vi "Main.vi"(8 "error in":errorcluster, 11 "CPU Percent in":refnum<class "CPU Percent.lvclass">) -> (0 "error out":errorcluster, 3 "CPU Percent out":refnum<class "CPU Percent.lvclass">)   [LabVIEW 2024, in "CPU Percent.lvclass"]
doc: "The <b>Queued Message Handler</b> of the Worker that owns this VI."
uses:
  CPU Percent.lvclass
  C:/Program Files (x86)/National Instruments/LabVIEW 2024/vi.lib/addons/_Workers/Library/Classes/Worker/Worker.lvclass
  CPU Percent.lvclass/CPU Percent.ctl
  rwr_Get CPU Percent Reply.ctl
  Controller/Controller.lvclass
  <vilib>/Analysis/baseanly.llb/Mean (DBL).vi
  <vilib>/Python/Open Venv Python Session.vi
  <vilib>/addons/_Workers/Library/Classes/Worker/Worker.lvclass
  <vilib>/addons/_Workers/Library/Classes/Message Queue/Message Queue.lvclass
  <vilib>/Analysis/NI_AALBase.lvlib
  Initialization Data.ctl
  C:/Program Files (x86)/National Instruments/LabVIEW 2024/vi.lib/addons/_Workers/Library/Classes/Workers Object/Workers Object.lvclass
  C:/_Repo/ugm24-dp2/src/Workers/CPU Percent/CPU Percent.lvclass
panel:
  out "CPU Core Percent":dbl[](array[numeric])
  out "Percent":dbl
  in  "GetPercent":bool
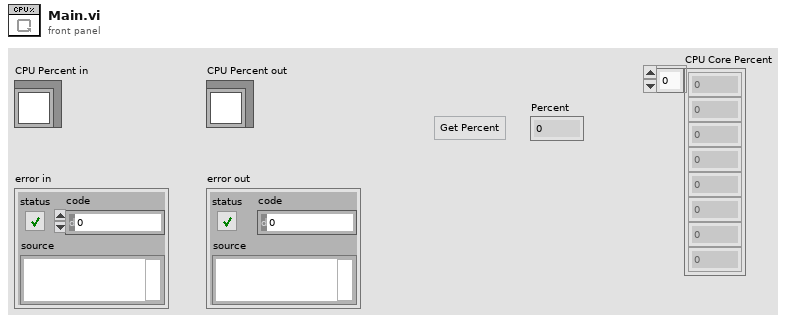
[diagram p1: front panel]
types:
  T1 = typedef "CPU Percent.lvclass/Initialization Data.ctl" = cluster{"String":string, "Show Frontpanel":bool}
  T2 = enum32{"Invalid", "Standard", "Closed", "Hidden", "Minimized", "Maximized"}
  T3 = typedef "CPU Percent.lvclass/rwr_Get CPU Percent Reply.ctl" = cluster{"Percent":dbl}
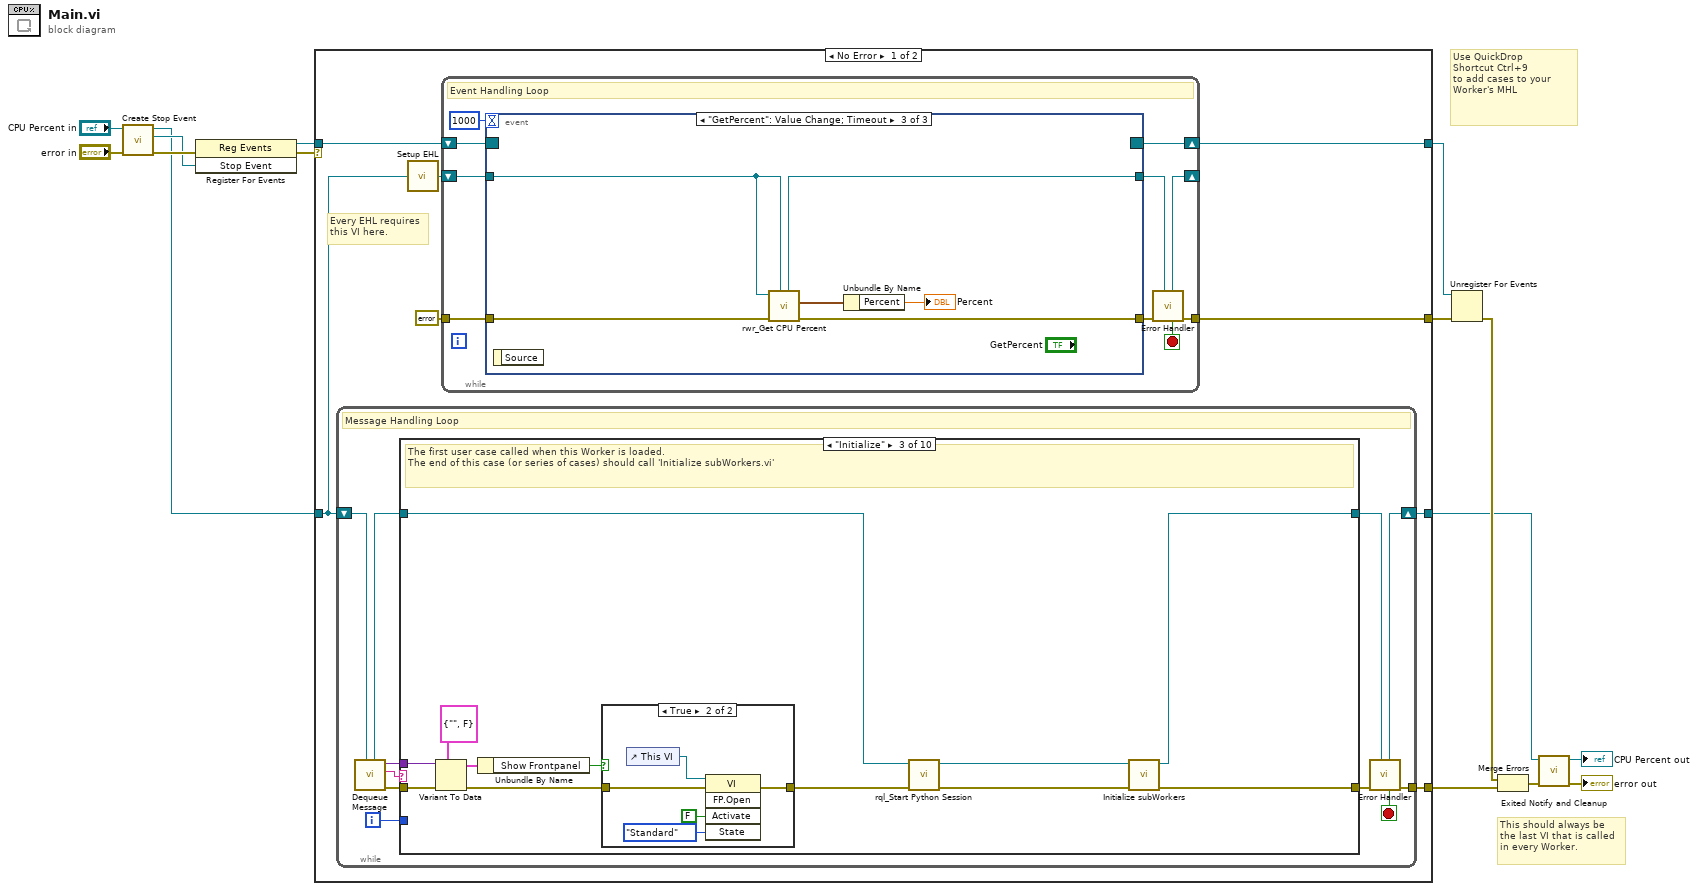
[diagram p0: block diagram]
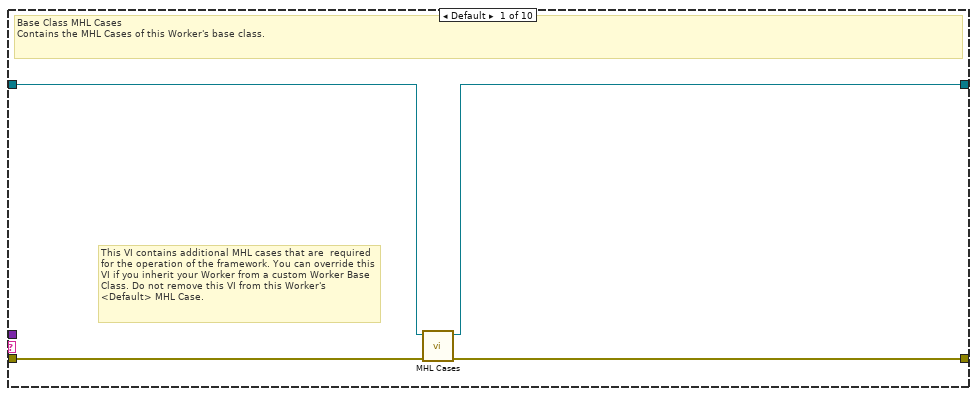
[diagram p2: hidden frame]
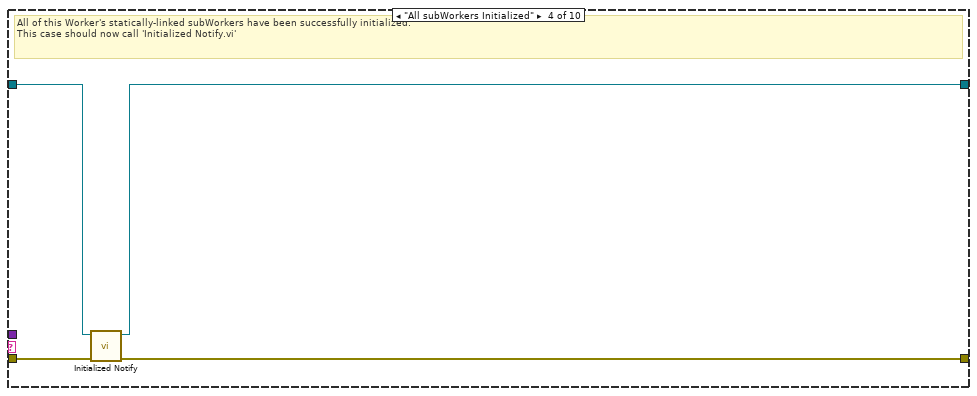
[diagram p5: hidden frame]
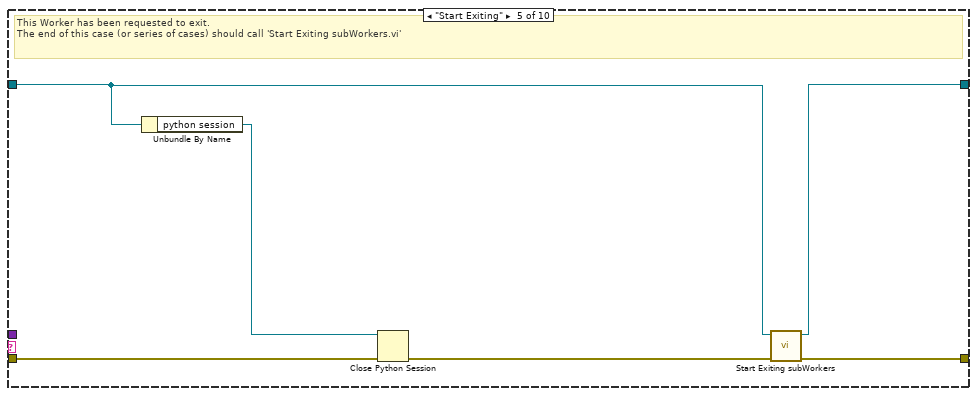
[diagram p6: hidden frame]
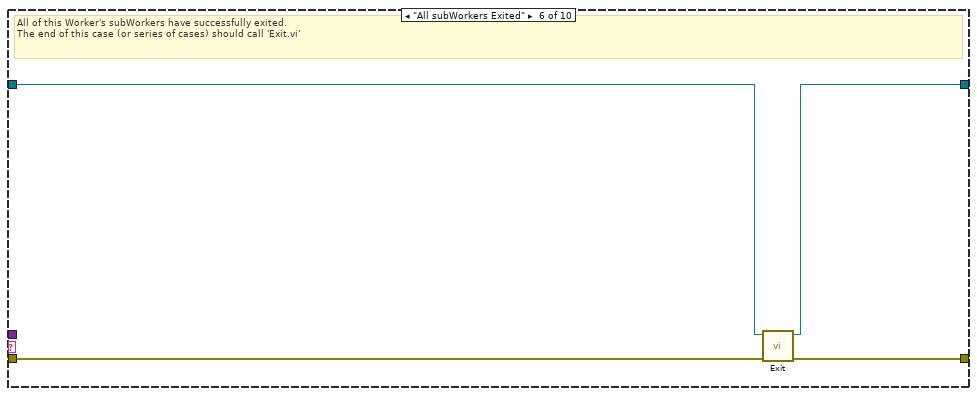
[diagram p7: hidden frame]
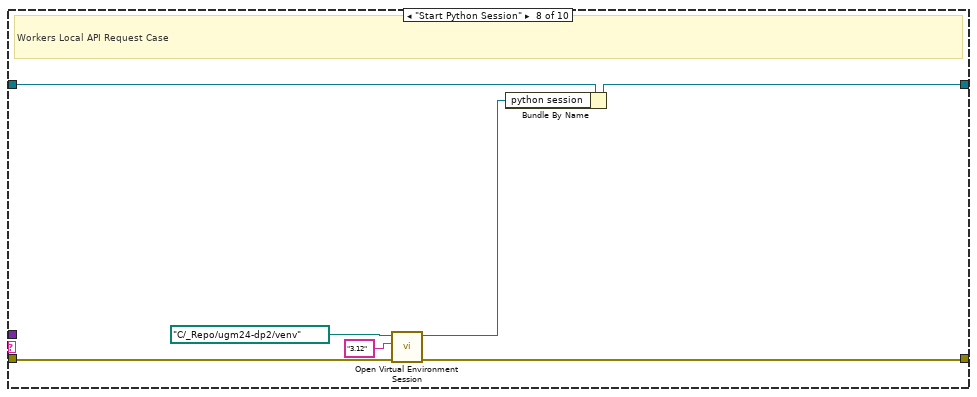
[diagram p9: hidden frame]
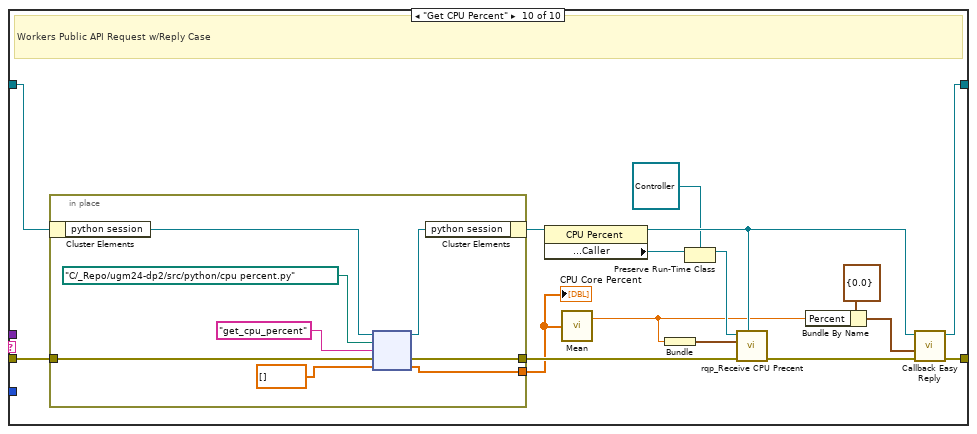
[diagram p11: hidden frame]
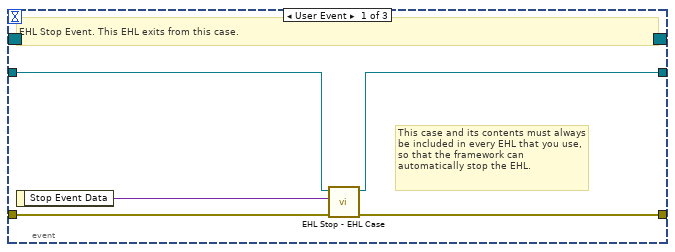
[diagram p12: hidden frame]
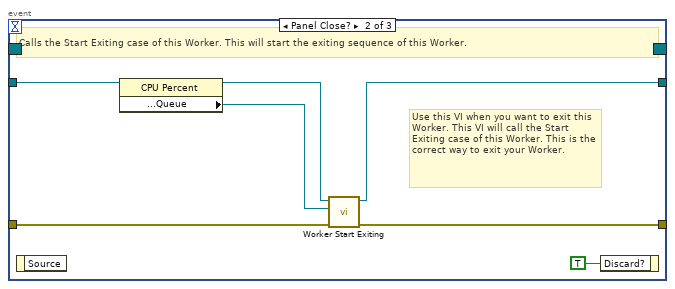
[diagram p13: hidden frame]
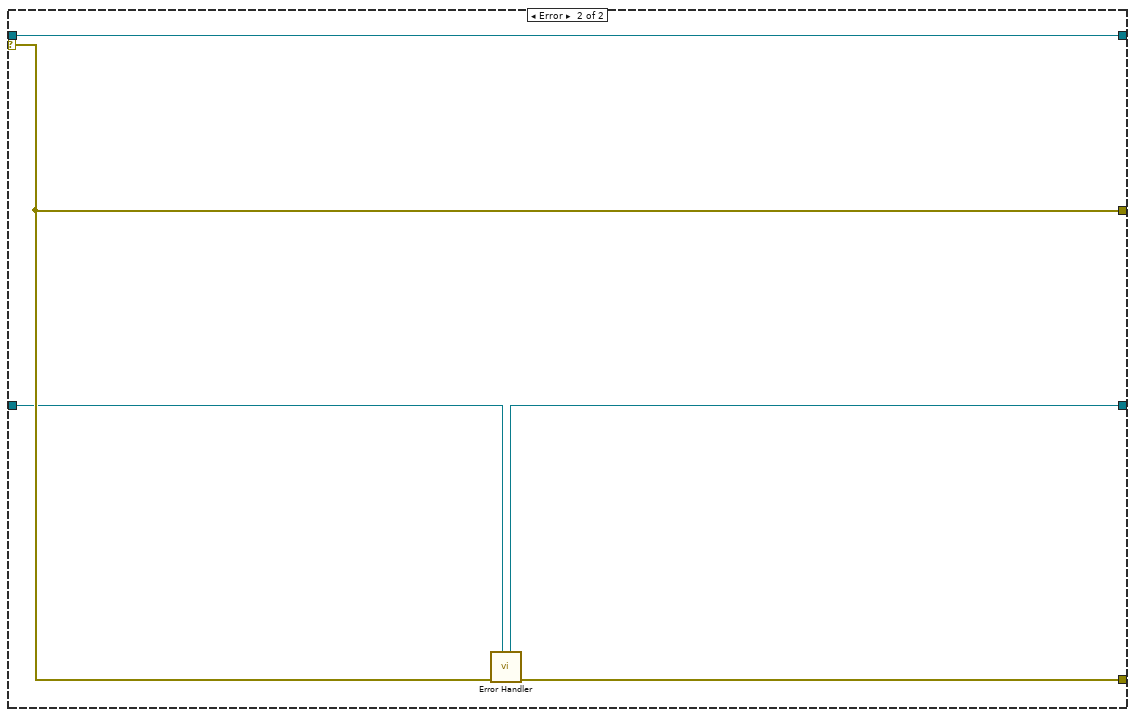
[diagram p14: hidden frame]
diagram:
  # "Use QuickDrop\nShortcut Ctrl+9\nto add cases to your\nWorker's MHL"
  # "This should always be the last VI that is called in every Worker."
  n1 = call-dynamic "Create Stop Event.vi"("error in"="error in", "Worker"="CPU Percent in") -> ("error out"=w10:errorcluster, "Stop Event"=w7:refnum<user-event>, "Worker out"=w4:refnum<class "CPU Percent.lvclass">)  [unwired: 7 in]
  n2 = register-events(error in=w10, w7) -> (reference out=w9:refnum<event-registration>, error out=w1:errorcluster)  [unwired: 1 in]
  n3 = case shown="No Error" w1 {
    tunnel: w4 -> [w18 w137]
    tunnel: [w16 w138] -> w8
    tunnel: w9 -> [w23 w139]
    tunnel: [w20 w140] -> w14
    tunnel: [w22 w139] -> w13
    tunnel: [w17 w136] -> w11
    selector: w1 -> [_ w140]
    frame No Error {
      # "Every EHL requires\nthis VI here."
      n4 = while {
        shift-right: [w32] -> w17
        shift-left: w18 -> [w34]
        tunnel: [w33] -> w16
        i -> [w25]
        stop <- w26 stop-if-true
        # "Message Handling Loop"
        n5 = call-dynamic "Dequeue Message.vi"("Worker"=w34) -> ("error out"=w31:errorcluster, "Case out"=w27:string, "Data out"=w24:variant, "Worker out"=w29:refnum<class "CPU Percent.lvclass">)  [unwired: 6 in, 1 out]
        n6 = case "Worker MHL Case Structure (DO NOT CHANGE LABEL NAME)" shown="\"Initialize\"" w27 {
          tunnel: w31 -> [w38 w39 w47 w60 w66 w72 w74 w78 w83 w96]
          tunnel: [w37 w39 w52 w59 w68 w71 w74 w77 w83 w99] -> w30
          tunnel: w29 -> [w36 w40 w48 w62 w65 w70 w73 w81 w82 w94]
          tunnel: [w35 w40 w51 w61 w67 w69 w73 w76 w82 w98] -> w28
          tunnel: w25 -> [_ _ _ _ _ _ _ _ _ _]
          tunnel: w24 -> [_ _ w45 _ _ _ _ _ _ _]
          frame Default {
            # "This VI contains additional MHL cases that are  required for the operation of the framework. You can override this VI if you inherit your Worker from a custom Worker Base Class. Do not remove this VI from this Worker's <Default> MHL Case."
            # "Base Class MHL Cases\nContains the MHL Cases of this Worker's base class."
            n7 = call-dynamic "MHL Cases.vi"("error in"=w38, "Worker in"=w36) -> ("error out"=w37:errorcluster, "Worker out"=w35:refnum<class "CPU Percent.lvclass">)  [unwired: 8 in]
          }
          frame "------------ FRAMEWORK CASES -----------" {
            # "Start of Workers Framework Cases"
          }
          frame "Initialize" {
            # "The first user case called when this Worker is loaded.\nThe end of this case (or series of cases) should call 'Initialize subWorkers.vi'"
            n8 = Variant To Data(error in=w47, type=T1 {"String"="", "Show Frontpanel"=FALSE} ("Initialization Data"), Variant=w45) -> (data=w42:T1, error out=w46:errorcluster)
            n9 = Unbundle By Name(w42) -> ("Show Frontpanel"=w41:bool)
            n10 = case shown="True" w41 {
              tunnel: w46 -> [w53 w58]
              tunnel: [w53 w57] -> w43
              frame False {
              }
              frame True {
                n11 = control-ref of="This VI"() -> (w56:refnum<vi>)
                n12 = invoke class="VI" method="FP.Open"(reference=w56, error in=w58, "Activate"=FALSE ("Activate?"), "State"=T2."Standard") -> (error out=w57:errorcluster)  [unwired: 1 in, 4 out]
              }
            }
            n13 = call "rql_Start Python Session.vi"("error in"=w43, "CPU Percent in"=w48) -> ("error out"=w50:errorcluster, "dup CPU Percent out"=w49:refnum<class "CPU Percent.lvclass">)  [unwired: 8 in]
            n14 = call-dynamic "Initialize subWorkers.vi"("error in"=w50, "Worker"=w49) -> ("error out"=w52:errorcluster, "dup Worker out"=w51:refnum<class "CPU Percent.lvclass">)  [unwired: 8 in]
          }
          frame "All subWorkers Initialized" {
            # "All of this Worker's statically-linked subWorkers have been successfully initialized.\nThis case should now call 'Initialized Notify.vi'"
            n15 = call-dynamic "Initialized Notify.vi"("error in"=w60, "Worker"=w62) -> ("error out"=w59:errorcluster, "dup Worker out"=w61:refnum<class "CPU Percent.lvclass">)  [unwired: 8 in]
          }
          frame "Start Exiting" {
            # "This Worker has been requested to exit. \nThe end of this case (or series of cases) should call 'Start Exiting subWorkers.vi'"
            n16 = Unbundle By Name(w65) -> ("python session"=w63:refnum<k35>)
            n17 = Close Python Session(session in=w63, error in=w66) -> (11:w64:errorcluster)
            n18 = call-dynamic "Start Exiting subWorkers.vi"("error_in"=w64, "Worker"=w65) -> ("error out"=w68:errorcluster, "dup Worker out"=w67:refnum<class "CPU Percent.lvclass">)  [unwired: 8 in]
          }
          frame "All subWorkers Exited" {
            # "All of this Worker's subWorkers have successfully exited. \nThe end of this case (or series of cases) should call 'Exit.vi'"
            n19 = call-dynamic "Exit.vi"("error_in"=w72, "Worker"=w70) -> ("error out"=w71:errorcluster, "dup Worker out"=w69:refnum<class "CPU Percent.lvclass">)  [unwired: 8 in]
          }
          frame "------------- LOCAL API CASES -------------" {
            # "Start of Workers Local API Cases"
          }
          frame "Start Python Session" {
            # "Workers Local API Request Case"
            n20 = call-poly <vilib>:"Open Virtual Environment Session.vi"("error in (no error)"=w78, "Python version"="3.12", "Env path"=path "C:/_Repo/ugm24-dp2/venv") -> ("error out"=w77:errorcluster, "session out"=w75:refnum<k35>)  [unwired: 7 in]
            n21 = Bundle By Name(cluster=w81, "python session"=w75) -> (w76:refnum<class "CPU Percent.lvclass">)
          }
          frame "------------- PUBLIC API CASES -------------" {
            # "Start of Workers Public API Cases"
          }
          frame "Get CPU Percent" {
            # "Workers Public API Request w/Reply Case"
            n22 = in-place {
              in-place-border: w96 -> [w107]
              in-place-border: [w101] -> w93
              in-place-border: [w100] -> w91
              n23 = in-place-cluster #1(w94) -> ("python session"=w106:refnum<k35>)
              n24 = node(w106, path "C:/_Repo/ugm24-dp2/src/python/cpu percent.py" ("module path"), "get_cpu_percent" ("function name"), w107, dbl[] []) -> (w105:refnum<k35>, w101:errorcluster, w100:dbl[])  [unwired: 2 out]
              n25 = in-place-cluster #1("python session"=w105) -> (w95:refnum<class "CPU Percent.lvclass">)
            }
            "CPU Core Percent" <- w91
            n26 = property class="CPU Percent"(reference=w95) -> (reference out=w89:refnum<class "CPU Percent.lvclass">, "Accessors:Read:Public API:Caller"=w88:refnum<class "Worker.lvclass">)  [unwired: 1 in, 1 out]
            n27 = call-poly <vilib>:"Mean.vi"("X"=w91) -> ("mean"=w85:dbl)  [unwired: 1 out]
            n28 = Bundle("mean"=w85) -> (w84:cluster{"mean":dbl})  [unwired: 1 in]
            n29 = Preserve Run-Time Class(object in=w88, 2:refnum<class "Controller.lvclass"> refnum ("Controller in")) -> (object out=w87:refnum<class "Controller.lvclass">)  [unwired: 1 in, 1 out]
            n30 = call "rqp_Receive CPU Precent.vi"("Caller in"=w89, "error in"=w93, "Data in"=w84, "Controller in"=w87) -> ("error out"=w90:errorcluster)  [unwired: 5 in, 2 out]
            n31 = Bundle By Name(cluster=T3 {"Percent"=0.0} ("Reply Data"), "Percent"=w85) -> (w92:T3)
            n32 = call-dynamic "Callback Easy Reply.vi"("error in"=w90, "Data"=w92, "Worker"=w89) -> ("error out"=w99:errorcluster, "dup Worker out"=w98:refnum<class "CPU Percent.lvclass">)  [unwired: 7 in]
          }
        }
        n33 = call-dynamic "Error Handler.vi"("Worker"=w28, "error_in"=w30) -> ("error out"=w33:errorcluster, "Stop Loop"=w26:bool, "Worker out"=w32:refnum<class "CPU Percent.lvclass">)  [unwired: 7 in]
      }
      n34 = call-dynamic "Setup EHL.vi"("Worker"=w18) -> ("Worker out"=w19:refnum<class "CPU Percent.lvclass">)  [unwired: 14 in]
      n35 = while "Event Handling Loop" {
        shift-right: [w117] -> w22
        shift-left: w23 -> [w116]
        tunnel: [w112] -> w20
        tunnel: errorcluster {"status"=FALSE, "code"=0, "source"=""} ("error constant") -> [w114]
        shift-right: [w110] -> _
        shift-left: w19 -> [w115]
        stop <- w109 stop-if-true
        # "Event Handling Loop"
        n36 = event shown="[2] \"GetPercent\": Value Change;  Timeout" {
          selector: w116 -> [_ _ _]
          dyn-events: [_ _ _] -> w117
          timeout: 1000 -> [_ _ _]
          tunnel: [w121 w128 w134] -> w113
          tunnel: w114 -> [w122 w127 w135]
          tunnel: w115 -> [w120 w126 w133]
          tunnel: [w119 w125 w132] -> w111
          event User Event {
            # "This case and its contents must always be included in every EHL that you use, so that the framework can automatically stop the EHL."
            # "EHL Stop Event. This EHL exits from this case."
            n37 = event-data() -> ("Stop Event Data"=w118:variant)  [unwired: 1 in]
            n38 = call-dynamic "EHL Stop - EHL Case.vi"("error in"=w122, "Stop Event Data"=w118, "Worker"=w120) -> ("error out"=w121:errorcluster, "Worker out"=w119:refnum<class "CPU Percent.lvclass">)  [unwired: 7 in]
          }
          event Panel Close? {
            # "Use this VI when you want to exit this Worker. This VI will call the Start Exiting case of this Worker. This is the correct way to exit your Worker."
            # "Calls the Start Exiting case of this Worker. This will start the exiting sequence of this Worker."
            n39 = event-data() -> ()  [unwired: 1 in, 1 out]
            n40 = property class="CPU Percent"(reference=w126) -> (reference out=w124:refnum<class "CPU Percent.lvclass">, "Accessors:Read:Public API:Queue"=w123:refnum<class "Message Queue.lvclass">)  [unwired: 1 in, 1 out]
            n41 = call-dynamic "Worker Start Exiting.vi"("error_in"=w127, "Message Queue"=w123, "Worker"=w124) -> ("error out"=w128:errorcluster, "dup Worker out"=w125:refnum<class "CPU Percent.lvclass">)  [unwired: 7 in]
            n42 = event-data("Discard?"=TRUE) -> ()  [unwired: 1 in, 1 out]
          }
          event "GetPercent": Value Change; Timeout {
            n43 = event-data() -> ()  [unwired: 1 in, 1 out]
            n44 = call "rwr_Get CPU Percent.vi"("Caller in"=w133, "error in"=w135, "CPU Percent in"=w133) -> ("error out"=w134:errorcluster, "Reply Data out"=w131:T3, "dup Caller out"=w132:refnum<class "CPU Percent.lvclass">)  [unwired: 5 in, 1 out]
            n45 = Unbundle By Name(w131) -> ("Percent"=→"Percent":dbl)
          }
        }
        n46 = call-dynamic "Error Handler.vi"("Worker"=w111, "error_in"=w113) -> ("error out"=w112:errorcluster, "Stop Loop"=w109:bool, "Worker out"=w110:refnum<class "CPU Percent.lvclass">)  [unwired: 7 in]
      }
    }
    frame Error {
      n47 = call-dynamic "Error Handler.vi"("Worker"=w137, "error_in"=w140) -> ("error out"=w138:errorcluster, "Worker out"=w136:refnum<class "CPU Percent.lvclass">)  [unwired: 7 in, 1 out]
    }
  }
  n48 = Unregister For Events(event registration refnum=w13, error in=w14) -> (error out=w15:errorcluster)
  n49 = Merge Errors(w15, w8) -> (w12:errorcluster)
  n50 = call-dynamic "Exited Notify and Cleanup.vi"("error_in"=w12, "Worker"=w11) -> ("error out"=→"error out":errorcluster, "dup Worker out"=→"CPU Percent out":refnum<class "CPU Percent.lvclass">)  [unwired: 8 in]
